vi "GenerateSyntheticData.vi"() -> ()   [LabVIEW 2011]
uses:
  BaesDataTypeDefinition.ctl
  <vilib>/Utility/file.llb/Write To Spreadsheet File (DBL).vi
  <vilib>/gmath/statdist.llb/Normal Inverse CDF.vi
  <vilib>/gmath/NI_Gmath.lvlib
panel:
  out "appended array":dbl[](array[numeric])
  out "Expected Extinction Cross Section":sgl[][](array[numeric])
  out "Concentration":dbl[][](array[numeric])
  out "Sizes":dbl[](array[numeric])
  out "GeometricCrossSection":dbl[](array[numeric])
  out "Number ofSizes":dbl
  out "Size parameters":dbl[](array[numeric])
  out "Numeric":i32
  out "size(s) 2":i32
  out "size(s)":i32
  in  "Population Size":i32=30
  in  "Extinction ExtinctionUncertainity Size parameter and Number ofS sizes":T1={"Extinction"=[], "Extinction Uncertainty"=[], "Size parameters"=[], "Number ofSizes"=0.0, "GeometricCrossSection"=[], "Wave Length"=0.0, "SMPS Sizes"=[], "Concentration"=[], "Double Charge Correction"=FALSE, "Extincation Factor"=1.0, "Diameter Factor"=1.0, "Diameter Offset"=0.0, "Extinction Factor Flag"=FALSE, "Diameter Factor Flag"=FALSE, "Diameter Offset Flag"=FALSE, "Sizes"=[]}
  in  "Extinction File 2":path=path "Z:/Dropbox/Lior Segev/Lior Segev Projects/RI retrieval in Labview/Data/SyntheticData/test.csv"
  out "Double Charge correction Initiated":bool=TRUE
  in  "Particle Concentration File":path=path "Z:/Dropbox/Lior Segev/Lior Segev Projects/RI retrieval in Labview/Data/SyntheticData/SRFA_Multiply charge distribution.txt"
  in  "Extinction File":path=path "Z:/Dropbox/Lior Segev/Lior Segev Projects/RI retrieval in Labview/Data/SyntheticData/SRFA_Spectrafit.csv"
  out "Number of Different Wavelengths":i32=130
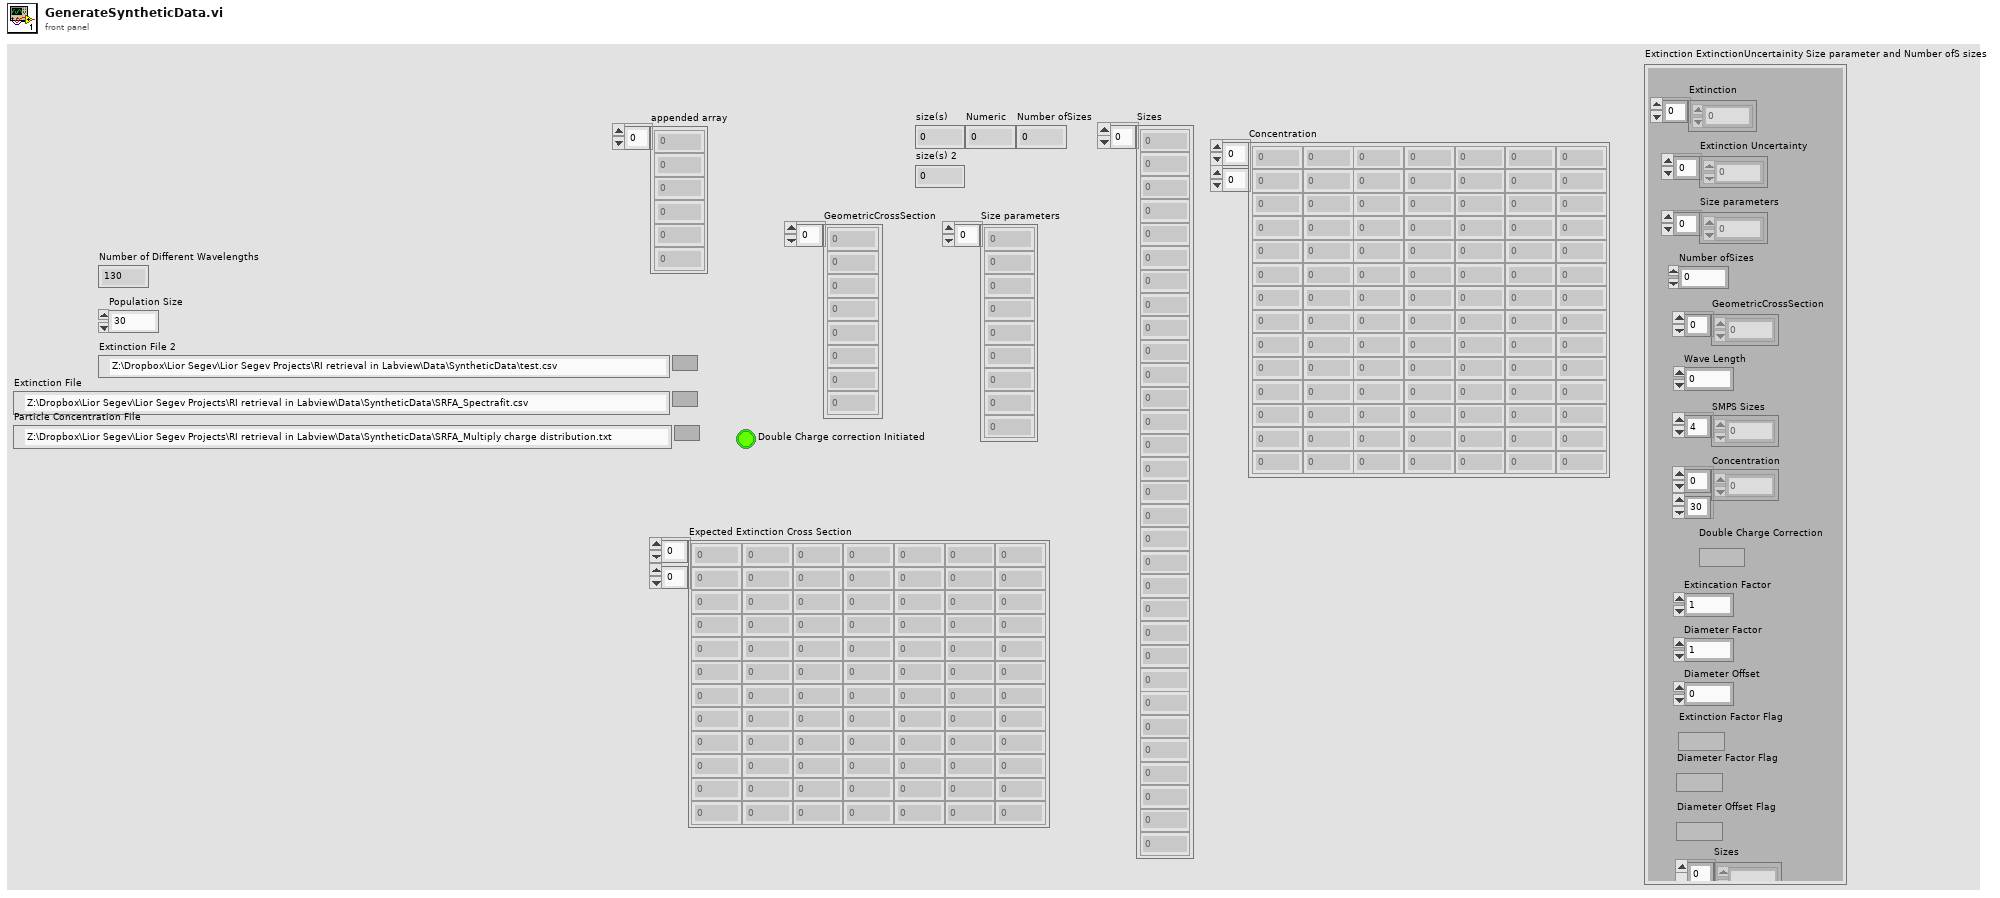
[diagram p1: front panel]
types:
  T1 = typedef "BaesDataTypeDefinition.ctl" = cluster{"Extinction":dbl[], "Extinction Uncertainty":dbl[], "Size parameters":dbl[], "Number ofSizes":dbl, "GeometricCrossSection":dbl[], "Wave Length":dbl, "SMPS Sizes":dbl[], "Concentration":dbl[][], "Double Charge Correction":bool, "Extincation Factor":dbl, "Diameter Factor":dbl, "Diameter Offset":dbl, "Extinction Factor Flag":bool, "Diameter Factor Flag":bool, "Diameter Offset Flag":bool, "Sizes":dbl[]}
  T2 = typedef "ReadBaesDataTypeDefinition.ctl" = cluster{"Extinction":dbl[][], "Extinction Uncertainty":dbl[][], "Size parameters":dbl[][], "Number ofSizes":dbl, "GeometricCrossSection":dbl[], "WaveLength":dbl[], "Sizes":dbl[]}
  T3 = typedef "ParticleDistributionData.ctl" = cluster{"SMPS Sizes":dbl[], "Concentration":dbl[][], "Double Charge Correction Flag":bool}
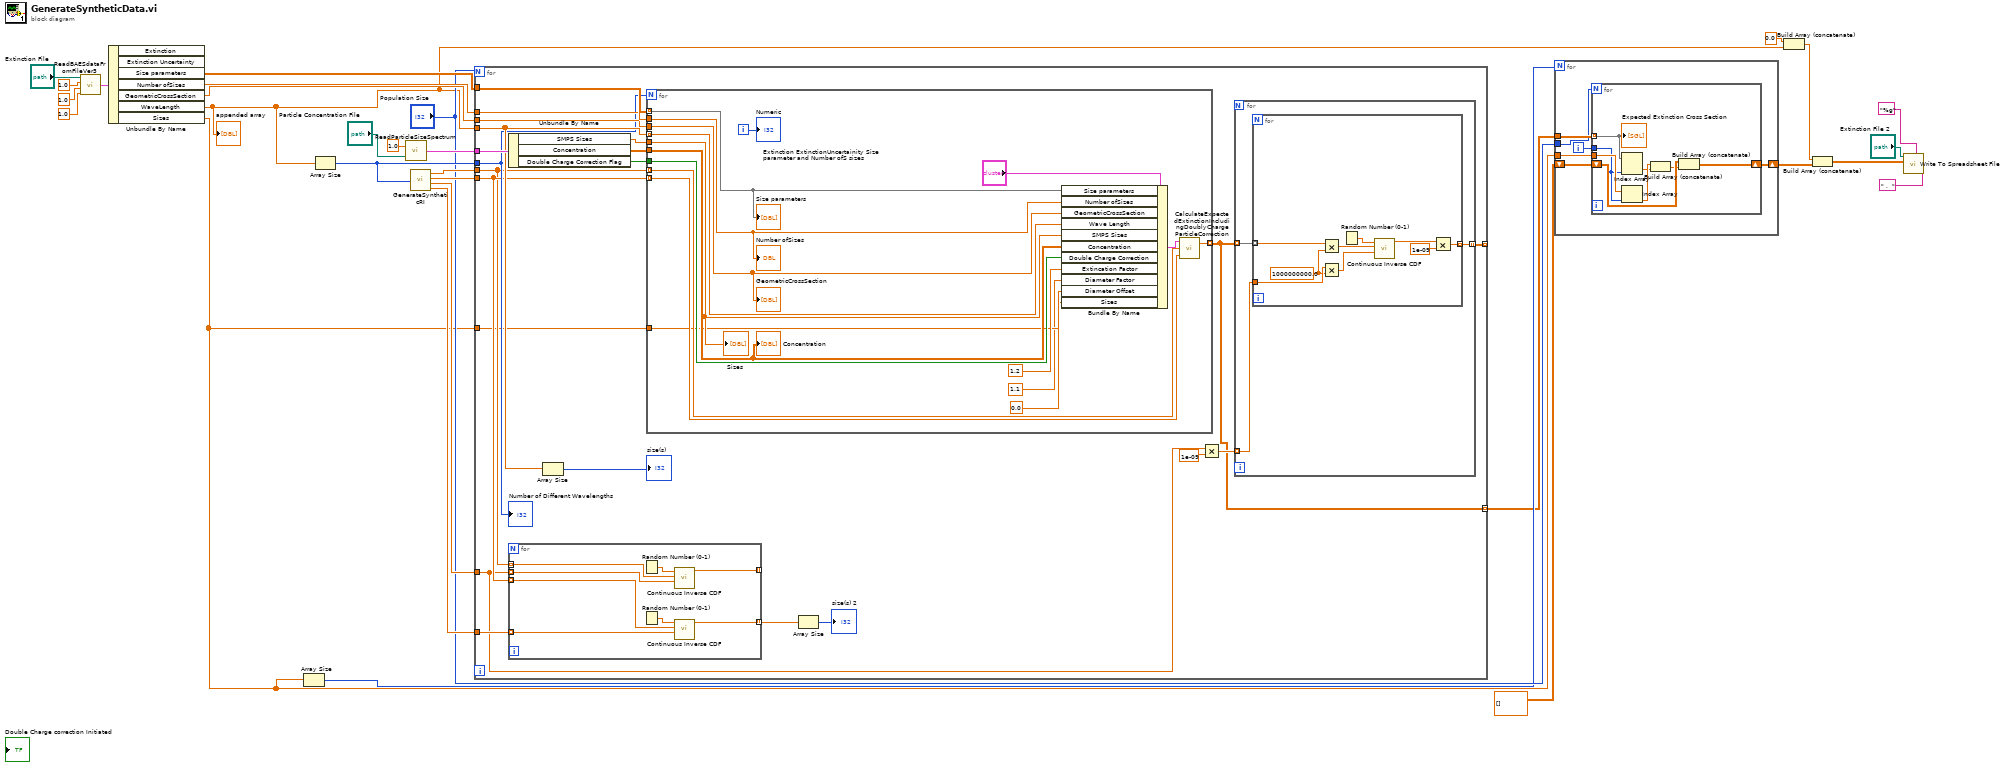
[diagram p0: block diagram]
diagram:
  n1 = call "ReadBAESdataFromFileVer3.vi"("Factor Size Parameter"=1.0, "Factor Extinction"=1.0, "Factor Ext Uncertainty"=1.0, "file path"="Extinction File") -> ("Extinction ExtinctionUncertainity Size parameter and Number ofS sizes"=w24:T2)
  n2 = Unbundle By Name(w24) -> ("Size parameters"=w22:dbl[][], "Number ofSizes"=w21:dbl, "GeometricCrossSection"=w20:dbl[], "WaveLength"=w8:dbl[], "Sizes"=w2:dbl[])  [unwired: 2 out]
  "appended array" <- w8
  n3 = Array Size(array=w2) -> (size(s)=w12:i32)
  n4 = Array Size(array=w8) -> (size(s)=w19:i32)
  n5 = call "ReadParticleSizeSpectrum.vi"("file path"="Particle Concentration File", "Factor Size paramter"=1.0) -> ("Particle Distribution Data"=w23:T3)
  n6 = call "GenerateSyntheticRI.vi"("Number of Wavelengths WL"=w19) -> ("Real Part per WL"=w18:dbl[], "Imaginary Part per WL"=w17:dbl[], "RealUncertainty"=w16:dbl[], "ImagiUncertainty"=w15:dbl[])
  n7 = for {
    N: "Population Size" -> [_]
    tunnel: w23 -> [w50]
    tunnel: w22 -> [w49]
    tunnel: w21 -> [w48]
    tunnel: w20 -> [w47]
    tunnel: w8 -> [w39]
    tunnel: w19 -> [w38]
    tunnel: w18 -> [w35]
    tunnel: w17 -> [w36]
    tunnel: w16 -> [w33]
    tunnel: w15 -> [w43]
    tunnel: [w37] -> _ mode=indexing
    tunnel: w2 -> [w31]
    tunnel: [w30] -> w1 mode=indexing
    n8 = Unbundle By Name(w50) -> ("SMPS Sizes"=w44:dbl[], "Concentration"=w46:dbl[][], "Double Charge Correction Flag"=w45:bool)
    n9 = for {
      tunnel: w35 -> [w69] mode=indexing
      tunnel: w33 -> [w68] mode=indexing
      tunnel: [w67] -> _ mode=indexing
      tunnel: w36 -> [w65] mode=indexing
      tunnel: w43 -> [w64] mode=indexing
      tunnel: [w63] -> w41 mode=indexing
      n10 = Random Number (0-1)() -> (number: 0 to 1=w70:dbl)
      n11 = Random Number (0-1)() -> (number: 0 to 1=w66:dbl)
      n12 = call-poly <vilib>:"Continuous Inverse CDF.vi"("std"=w68, "mean"=w69, "cdf(x)"=w70) -> ("x"=w67:dbl)  [unwired: 7 in, 1 out]
      n13 = call-poly <vilib>:"Continuous Inverse CDF.vi"("std"=w64, "mean"=w65, "cdf(x)"=w66) -> ("x"=w63:dbl)  [unwired: 7 in, 1 out]
    }
    n14 = Array Size(array=w39) -> (size(s)=→"size(s)":i32)
    n15 = for {
      N: w38 -> [_]
      tunnel: w35 -> [w87] mode=indexing
      tunnel: w36 -> [w86] mode=indexing
      tunnel: [w85] -> w30 mode=indexing
      tunnel: w49 -> [w82] mode=indexing
      tunnel: w48 -> [w81]
      tunnel: w47 -> [w80]
      tunnel: w39 -> [w79] mode=indexing
      tunnel: w44 -> [w78]
      tunnel: w46 -> [w77]
      tunnel: w45 -> [w76]
      tunnel: w31 -> [w72]
      i -> [w75]
      n16 = Bundle By Name(cluster="Extinction ExtinctionUncertainity Size parameter and Number ofS sizes", "Size parameters"=w82, "Number ofSizes"=w81, "GeometricCrossSection"=w80, "Wave Length"=w79, "SMPS Sizes"=w78, "Concentration"=w77, "Double Charge Correction"=w76, "Extincation Factor"=1.2, "Diameter Factor"=1.1, "Diameter Offset"=0.0, "Sizes"=w72) -> (w83:T1)
      n17 = call "CalculateExpectedExtinctionIncludingDoublyChargeParticleCorrection.vi"("refractive index, imaginary"=w86, "refractive index, real"=w87, "Extinction ExtinctionUncertainity Size parameter and Number ofS sizes"=w83) -> ("Expected Extinction Cross Section"=w85:sgl[])  [unwired: 1 out]
      "Numeric" <- w75
      "Size parameters" <- w82
      "Number ofSizes" <- w81
      "GeometricCrossSection" <- w80
      "Sizes" <- w78
      "Concentration" <- w77
    }
    n18 = Array Size(array=w41) -> (size(s)=→"size(s) 2":i32)
    n19 = Multiply(x=w33, y=1e-09) -> (x*y=w34:dbl[])
    n20 = for {
      tunnel: w30 -> [w53] mode=indexing
      tunnel: w34 -> [w52] mode=indexing
      tunnel: [w51] -> w37 mode=indexing
      n21 = for {
        tunnel: w53 -> [w61] mode=indexing
        tunnel: w52 -> [w59]
        tunnel: [w54] -> w51 mode=indexing
        w58 = 1000000000.0 ("y")
        n22 = Multiply(x=w61, y=w58) -> (x*y=w60:dbl)
        n23 = Multiply(x=w59, y=w58) -> (x*y=w57:dbl)
        n24 = Random Number (0-1)() -> (number: 0 to 1=w62:dbl)
        n25 = call-poly <vilib>:"Continuous Inverse CDF.vi"("std"=w57, "mean"=w60, "cdf(x)"=w62) -> ("x"=w56:dbl)  [unwired: 7 in, 1 out]
        n26 = Multiply(x=w56, y=1e-09) -> (x*y=w54:dbl)
      }
    }
    "Number of Different Wavelengths" <- w38
  }
  n27 = for {
    N: w12 -> [_]
    tunnel: w1 -> [w93]
    tunnel: "Population Size" -> [w91]
    tunnel: w2 -> [w90]
    shift-right: [w89] -> w10
    shift-left: sgl[][] [] ("Expected Extinction Cross Section") -> [w92]
    i -> [w88]
    n28 = for {
      N: w91 -> [_]
      tunnel: w93 -> [w99] mode=indexing
      shift-right: [w100] -> w89
      shift-left: w92 -> [w101]
      tunnel: w90 -> [w98]
      tunnel: w88 -> [w94]
      n29 = Index Array(array=w99, index (col)=w94) -> (element=w96:sgl[])  [unwired: 1 in]
      n30 = Index Array(array=w98, index=w94) -> (element=w97:dbl)
      n31 = Build Array (concatenate)(w97, w96) -> (w95:dbl[])
      n32 = Build Array (concatenate)(w101, w95) -> (w100:dbl[][])
      "Expected Extinction Cross Section" <- w99
    }
  }
  n33 = Build Array (concatenate)(0.0 ("element"), w8) -> (w7:dbl[])
  n34 = Build Array (concatenate)(w7, w10) -> (w9:dbl[][])
  n35 = call-poly <vilib>:"Write To Spreadsheet File.vi"("delimiter (\\t)"=" ,  " ("delimiter (\\t)"), "format (%.3f)"="%g", "2D data"=w9, "file path (dialog if empty)"="Extinction File 2") -> ()  [unwired: 4 in, 1 out]
